vi "Automation.vi"   [LabVIEW 2015]
uses:
  AutomationDriveStates.ctl
  ArmStates.ctl
  <vilib>/Rock Robotics/WPI/Solenoid/WPI_SolenoidValue.ctl
  Robot Global Data.vi
  <vilib>/Rock Robotics/Network Tables/NT Read String.vi
  <vilib>/Rock Robotics/WPI/Solenoid/WPI_SolenoidSetEnum.vi
  <vilib>/addons/control/pid/pid.llb/PID (DBL).vi
  navX-MXP Library/navX-MXP IMU.lvlib
  <vilib>/addons/control/pid/NI_PID_pid.lvlib
types:
  T1 = typedef "AutomationDriveStates.ctl" = enum16{"Find Target", "Just Drive", "Nothing", "Moat", "Rockwall", "Drawbridge Defense", "Drawbridge Drive", "Advance To Defense", "Check Defense Type", "Drive Over Defense", "Stop Drives", "Advance To Target", "Move Forward", "Turn Mid Y", "Move Mid Y", "Center Target"}
  T2 = typedef "ArmStates.ctl" = enum16{"Arm Drive Position", "Winch Up", "Level Arm", "Hold Climb", "Drawbridge Drive Forward", "Shoot Position", "Roll Out", "Hic Up Rollers Off", "Draw Bridge Arm Down", "Harvest Back Down", "Harvest Hic up", "Portcullis", "Sally Door", "Harvest", "Arm Up", "Arm Down"}
  T3 = typedef "WPI_SolenoidValue.ctl" = enum16{"Off", "On", "Forward", "Reverse"}
  T4 = cluster{"proportional gain (Kc)":dbl, "integral time (Ti, min)":dbl, "derivative time (Td, min)":dbl}
  T5 = cluster{"Direction (T=CW)":bool, "Target Left Pos":dbl, "Target Right Pos":dbl, "Target Width":dbl, "Target Center":dbl, "Target Distance from Right":dbl, "Left Drive Speed":dbl, "Right Drive Speed":dbl, "System State":T1, "Lost Target Counter":dbl, "Last Drive Time":u32, "Distance From Target":dbl, "Starting Heading":dbl, "Current Heading":dbl, "Delta Heading":dbl, "Initial Diustance to Target":dbl, "Starting Encoder Position":dbl, "Current Encoder Position":dbl, "Encoder Counts Per Real Ft":dbl, "Encoder Count Per Calc Ft":dbl, "Starting Calc Distance":dbl, "Starting Left Position":dbl, "Starting Right Position":dbl, "Target Angle":dbl, "Target Distance":dbl, "In Position?":bool, "Desired Arm State":T2, "Shoot":bool, "Spin Up Shooter Wheels":bool, "Right of Target":bool, "Drive To Defense Counter":u32}
  T6 = typedef "WPI_MotorControlDeviceRef.ctl" = cluster{"DeviceStatus":errorcluster, "Type":T7, "PWM":cluster{"PWM Channel":T8, "DeadBand":T9}, "CAN":cluster{"Device Number":u8, "Control Mode":T10, "Semaphore":T11, "Max Vout":dbl, "TalonSRX Control Mode":T12}, "Invert":bool}
  T7 = typedef "WPI_MotorControlType.ctl" = enum16{"PWM", "CAN", "CANTalonSRX"}
  T8 = typedef "FPGA_DIOPWMChannel.ctl" = enum8{"PWM 0", "PWM 1", "PWM 2", "PWM 3", "PWM 4", "PWM 5", "PWM 6", "PWM 7", "PWM 8", "PWM 9", "PWM MXP 0", "PWM MXP 1", "PWM MXP 2", "PWM MXP 3", "PWM MXP 4", "PWM MXP 5", "PWM MXP 6", "PWM MXP 7", "PWM MXP 8", "PWM MXP 9", "Invalid"}
  T9 = typedef "WPI_PWMDeadband.ctl" = cluster{"Name":string, "maxPositivePwm":i32, "minPositivePwm":i32, "centerPwm":i32, "maxNegativePwm":i32, "minNegativePwm":i32, "angularRange":u16}
  T10 = typedef "WPI_CANJaguar_ControlMode.ctl" = enum8{"Percent VBus", "Current", "Speed", "Position", "Voltage"}
  T11 = typedef "Semaphore RefNum" = refnum<k1>
  T12 = typedef "WPI_CANTalonSRX_APIControlMode.ctl" = enum8{"Percent VBus", "Speed", "Position", "Slave", "Unchanged / Invalid", "Voltage Compensation", "Current", "Motion Profile"}
  T13 = typedef "navX-MXP IMU.lvlib/navX Device TypeDef.ctl" = cluster{"navX Interface Protocol":T14, "navX Interface Protocol TypeDefs":cluster{"SPIDevRef":T15, "I2CDevRef":T17}, "navX System Information":cluster{"Board Information":T19, "Status":T22, "Offsets":T26, "LastSampleTimestamp":dbl, "LastSampleValid":bool}, "navX Common Information":cluster{"Update Rate (4Hz-60Hz)":T27, "refnum name":string, "error":errorcluster, "LastSampleFPGATimestamp":dbl}}
  T14 = typedef "navX-MXP IMU.lvlib/navX Interface Protocol.ctl" = enum16{"SPI", "I2C", "SERIAL"}
  T15 = typedef "WPI_SPIDevRef.ctl" = cluster{"DevStatus":errorcluster, "Handle":i32, "SPI Bus":T16}
  T16 = typedef "spi_bus.ctl" = enum16{"SPI On-Board, CS0", "SPI On-Board, CS1", "SPI On-Board, CS2", "SPI On-Board, CS3", "SPI MXP", "Invalid"}
  T17 = typedef "WPI_I2CDevRef.ctl" = cluster{"DevStatus":errorcluster, "Device Address":u8, "Handle":i32, "I2C Bus":T18}
  T18 = typedef "i2c_bus.ctl" = enum16{"I2C On-Board", "I2C MXP", "Invalid"}
  T19 = typedef "navX-MXP IMU.lvlib/navX Board Information.ctl" = cluster{"WhoAmI (50 | 0x32)":u8, "Board Revision":u8, "Firmware Major Version":u8, "Firmware Minor Version":u8, "NAVX_BOARD_CAPABILITY":T20, "NAVX_BOARD_YAW_AXIS":T21}
  T20 = typedef "navX-MXP IMU.lvlib/navX NAVX_BOARD_CAPABILITY.ctl" = cluster{"OMNIMOUNT":bool, "YAW_RESET":bool, "VEL_AND_DISP":bool}
  T21 = typedef "navX-MXP IMU.lvlib/navX NAVX_BOARD_YAW_AXIS.ctl" = cluster{"BOARD_YAW_AXIS_UP":bool, "BOARD_YAW_AXIS":u8}
  T22 = typedef "navX-MXP IMU.lvlib/navX Status Data.ctl" = cluster{"Update Rate Hz":u8, "Accelerometer Full-Scale Range":u8, "Gyro Full-Scale Range":u16, "NAVX_OP_STATUS":T23, "NAVX_CAL_STATUS":T24, "NAVX_SELFTEST_STATUS":u8, "NAVX_SENSOR_STATUS":T25}
  T23 = typedef "navX-MXP IMU.lvlib/navX NAVX_OP_STATUS.ctl" = u8
  T24 = typedef "navX-MXP IMU.lvlib/navX NAVX_CAL_STATUS.ctl" = u8
  T25 = typedef "navX-MXP IMU.lvlib/navX NAVX_SENSOR_STATUS.ctl" = cluster{"MOVING":bool, "YAW_STABLE":bool, "MAG_DISTURBANCE":bool, "ALTITUDE_VALID":bool, "SEALEVEL_PRESS_SET":bool, "FUSED_HEADING_VALID":bool}
  T26 = typedef "navX-MXP IMU.lvlib/navX Offsets Data.ctl" = cluster{"Yaw":dbl, "Quat W":dbl, "Quat X":dbl, "Quat Y":dbl, "Quat Z":dbl}
  T27 = typedef "navX-MXP IMU.lvlib/navX Update Rate.ctl" = u8
  T28 = typedef "WPI_CANTalonSRX_GlobalStatus.ctl" = cluster{"Applied Throttle":dbl, "Module Enabled":bool, "CAN Error":errorcluster, "Closed Loop Error":dbl, "Forward Limit Switch Closed":bool, "Reverse Limit Switch Closed":bool, "Sensor Position":dbl, "Sensor Velocity":dbl, "Current":dbl, "Sticky Fault - Over Temp":bool, "Sticky Fault - Under Voltage":bool, "Sticky Fault - Forward Limit":bool, "Sticky Fault - Reverse Limit":bool, "Sticky Fault - Forward Soft Limit":bool, "Sticky Fault - Reverse Soft Limit":bool, "Brake is Enabled":bool, "Encoder Position":dbl, "Encoder Velocity":dbl, "Encoder Index Count":dbl, "Encoder A Pin State":bool, "Encoder B Pin State":bool, "Encoder Index Pin State":bool, "Analog In":dbl, "Analog In Velocity":dbl, "Temperature (C)":dbl, "Battery Voltage":dbl, "Control 5 Is Supported":bool, "Current Profile Slot Select":dbl, "Pos Div 8":bool, "Vel Div 4":bool, "Pulse Width Position":i32, "Pulse Width Velocity":i32, "Pulse Width Rise To Rise (us)":i32, "Pulse Width Rise To Fall (us)":i32, "Mot Prof Active Is Under Run":bool, "Mot Prof Active Has Under Run":bool, "Mot Prof Active Is Last":bool, "Mot Prof Active Velocity Only":bool, "Mot Prof Active Is Valid":bool, "Mot Prof Buffer Is Full":bool, "Mot Prof Active Profile Slot Select":i32, "Mot Prof NextID":i32, "Mot Prof Count":i32, "Mot Prof Active Velocity":dbl, "Mot Prof Active Position":dbl, "Mot Prof Output Enable":i32}
  T29 = typedef "navX-MXP IMU.lvlib/navX YPRH Data.ctl" = cluster{"Yaw":dbl, "Pitch":dbl, "Roll":dbl, "Heading":dbl}
  T30 = typedef "WPI_SolenoidDevRef.ctl" = cluster{"DevStatus":errorcluster, "Pneumatics Control Module":u8, "Forward Solenoid Channel":T31, "Reverse Solenoid Channel":T31}
  T31 = typedef "WPI_SolenoidChannel.ctl" = enum8{"Solenoid 0", "Solenoid 1", "Solenoid 2", "Solenoid 3", "Solenoid 4", "Solenoid 5", "Solenoid 6", "Solenoid 7", "Invalid"}
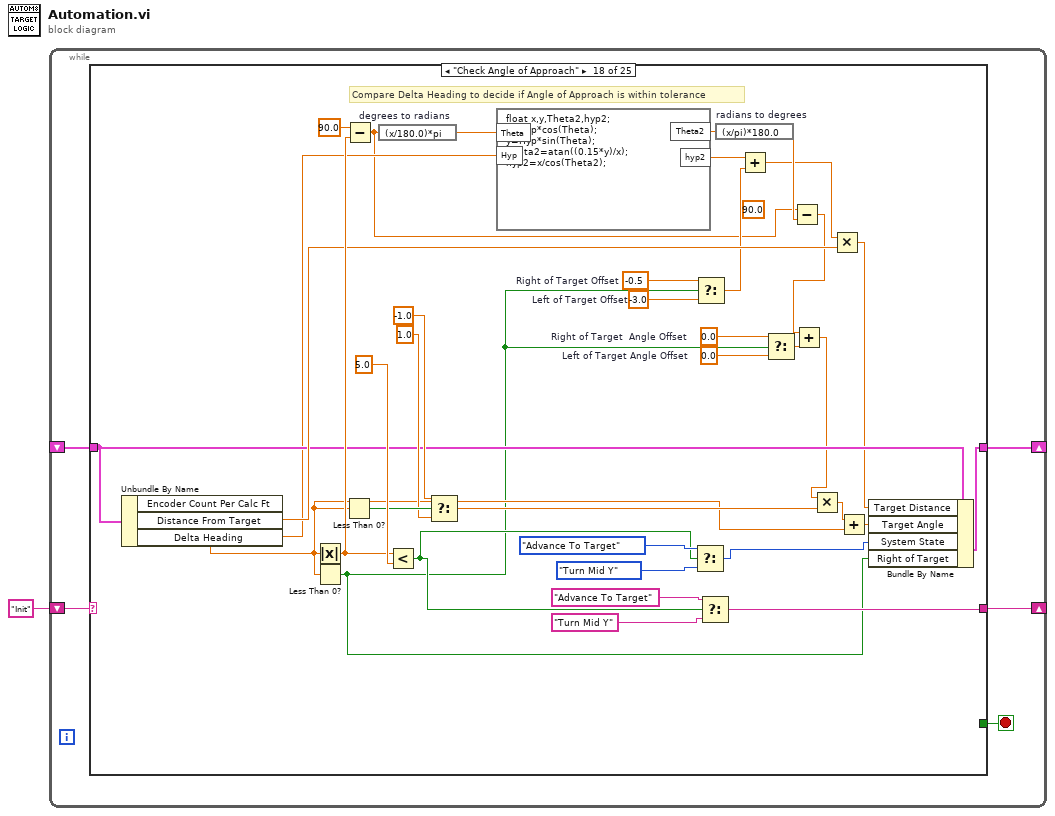
[diagram p0: block diagram]
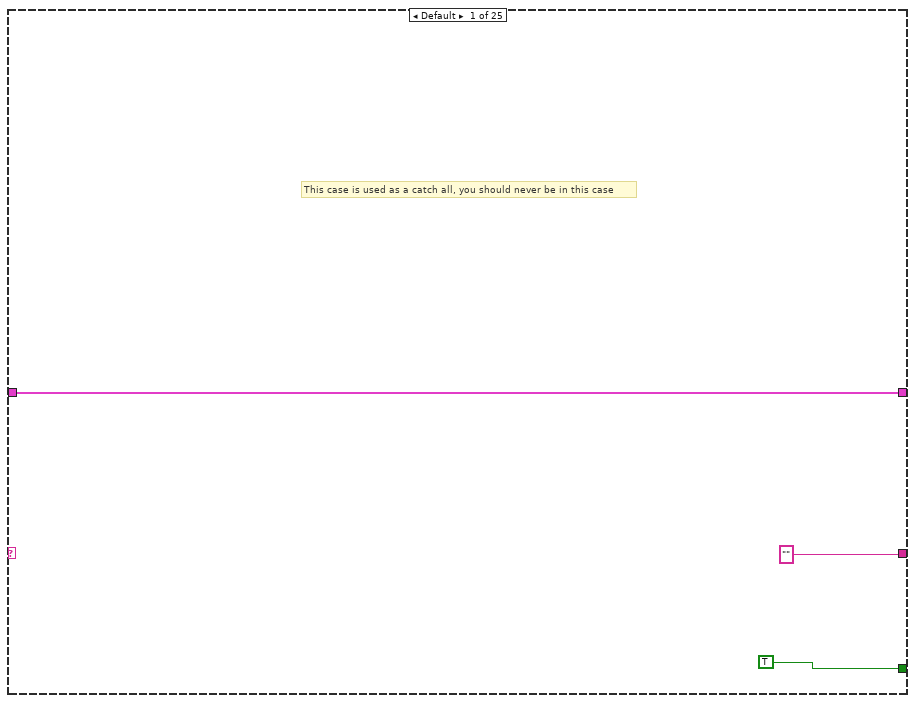
[diagram p2: hidden frame]
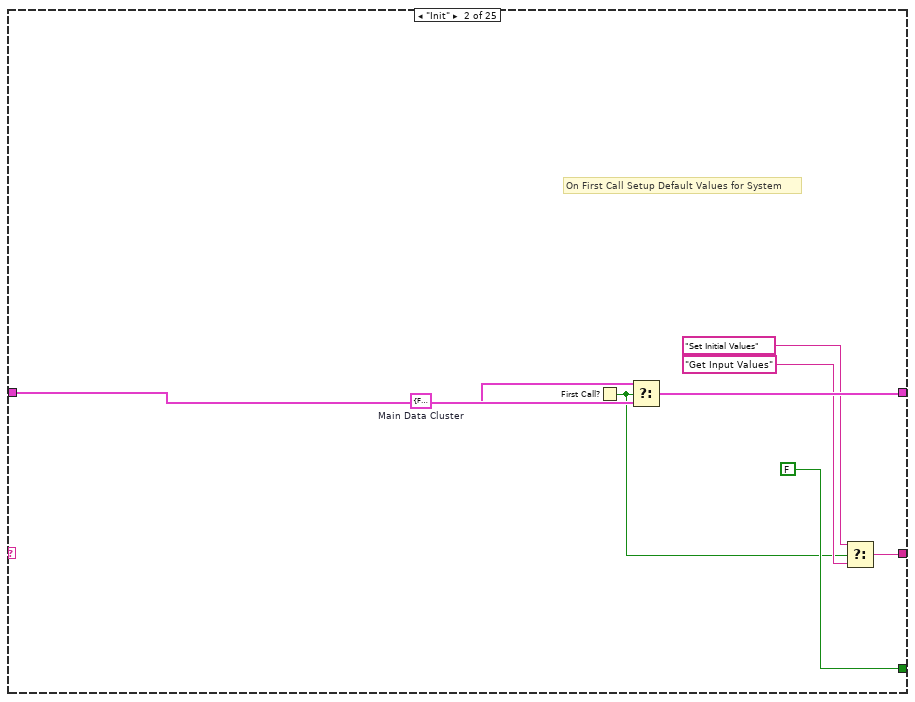
[diagram p3: hidden frame]
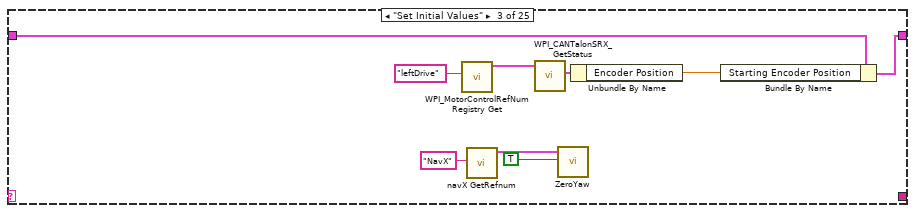
[diagram p4: hidden frame]
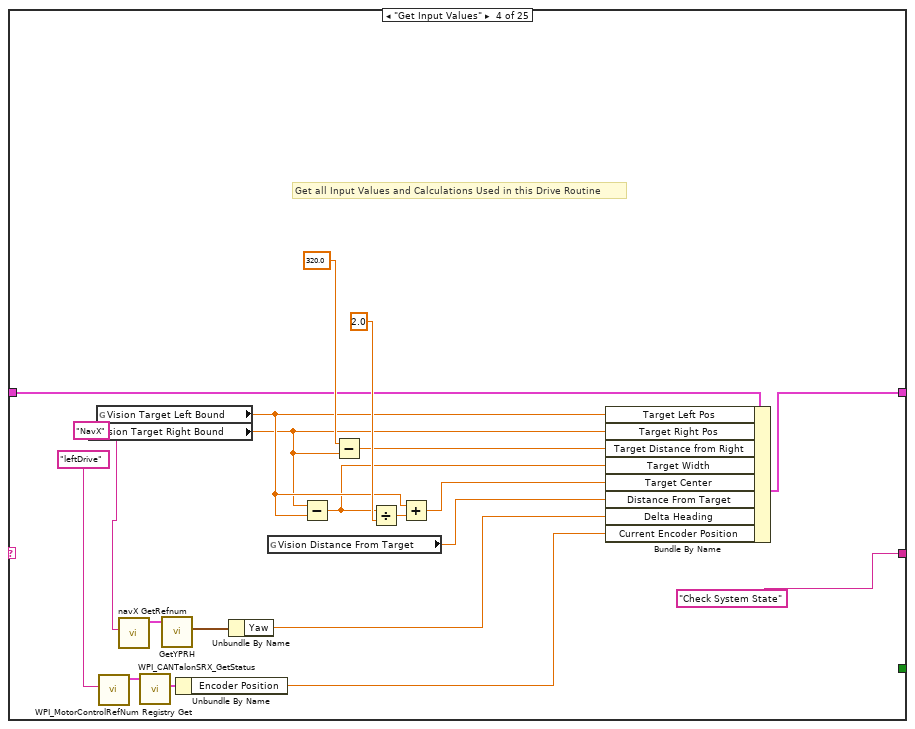
[diagram p5: hidden frame]
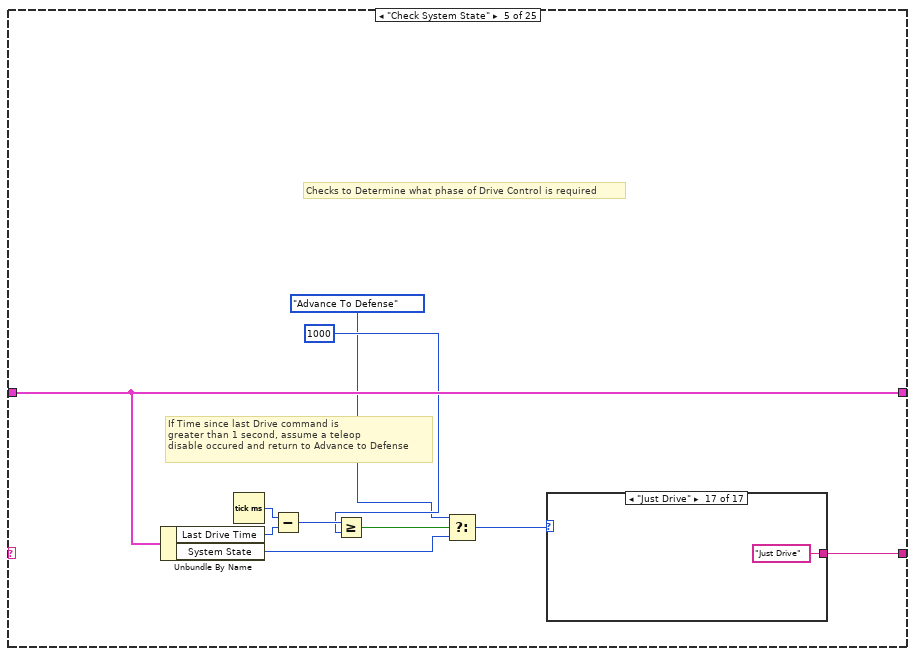
[diagram p6: hidden frame]
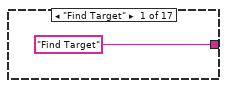
[diagram p7: hidden frame]
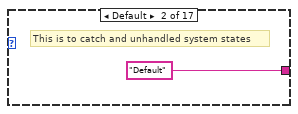
[diagram p8: hidden frame]
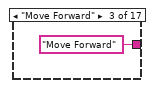
[diagram p9: hidden frame]
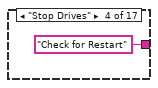
[diagram p10: hidden frame]
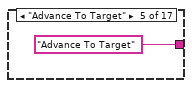
[diagram p11: hidden frame]
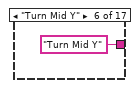
[diagram p12: hidden frame]
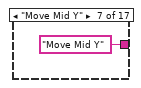
[diagram p13: hidden frame]
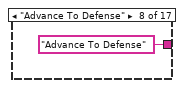
[diagram p14: hidden frame]
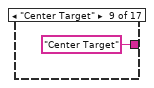
[diagram p15: hidden frame]
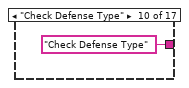
[diagram p16: hidden frame]
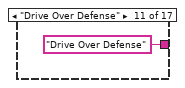
[diagram p17: hidden frame]
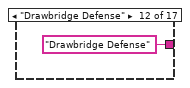
[diagram p18: hidden frame]
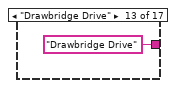
[diagram p19: hidden frame]
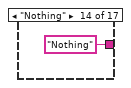
[diagram p20: hidden frame]
diagram:
  n1 = while {
    shift-right: [w6] -> _
    shift-left: "Init" -> [w2]
    shift-right: [w5] -> _
    shift-left: _ -> [w4]
    stop <- w3 stop-if-true
    n2 = case shown="\"Check Angle of Approach\"" w2 {
      tunnel: ["" w10 _ "Check System State" w55 w75 w108 w127 w144 "Drive Motors" w166 w183 w197 w215 w248 "Drive Motors" w287 w330 w343 w366 "Check for Stop" w407 "Exit" "Exit" _] -> w6
      tunnel: [w9 w14 w25 w43 w56 w102 w113 w135 w152 w157 w174 w191 w206 w210 w254 w277 w299 w329 w355 w374 w403 w411 w438 w483 w500] -> w5
      tunnel: w4 -> [w9 w16 w26 w36 w56 w100 w112 w133 w150 w155 w172 w189 w193 w211 w255 w278 w297 w318 w356 w372 w404 w412 w437 w484 w500]
      tunnel: [TRUE FALSE _ _ _ _ _ _ _ _ _ _ _ _ _ _ _ _ _ _ _ _ _ _ TRUE] -> w3
      frame Default {
        # "This case is used as a catch all, you should never be in this case"
      }
      frame "Init" {
        w15 = T5 {"Direction (T=CW)"=FALSE, "Target Left Pos"=0.0, "Target Right Pos"=0.0, "Target Width"=0.0, "Target Center"=0.0, "Target Distance from Right"=0.0, "Left Drive Speed"=0.0, "Right Drive Speed"=0.0, "System State"=enum."Advance To Defense", "Lost Target Counter"=0.0, "Last Drive Time"=0, "Distance From Target"=0.0, "Starting Heading"=0.0, "Current Heading"=0.0, "Delta Heading"=0.0, "Initial Diustance to Target"=0.0, "Starting Encoder Position"=0.0, "Current Encoder Position"=0.0, "Encoder Counts Per Real Ft"=0.0, "Encoder Count Per Calc Ft"=0.0, "Starting Calc Distance"=0.0, "Starting Left Position"=0.0, "Starting Right Position"=0.0, "Target Angle"=0.0, "Target Distance"=0.0, "In Position?"=FALSE, "Desired Arm State"=enum."Arm Drive Position", "Shoot"=FALSE, "Spin Up Shooter Wheels"=FALSE, "Right of Target"=FALSE, "Drive To Defense Counter"=0}  # Main Data Cluster
        # "On First Call Setup Default Values for System"
        n3 = First Call?() -> (First Call?: T/F=w11:bool)
        n4 = Select(t=w15, s=w11, f=w16) -> (s? t:f=w14:T5)
        n5 = Select(t="Set Initial Values", s=w11, f="Get Input Values") -> (s? t:f=w10:string)
      }
      frame "Set Initial Values" {
        n6 = call <vilib>:"WPI_MotorControlRefNum Registry Get.vi"("refnum name"="leftDrive") -> ("MotorControlDevRef"=w24:T6)  [unwired: 9 in, 1 out]
        n7 = call "navX GetRefnum.vi"("refnum name"="NavX") -> ("navX Device TypeDef"=w20:T13)  [unwired: 9 in, 1 out]
        n8 = call <vilib>:"WPI_CANTalonSRX_GetStatus.vi"("CAN Talon SRX Ref"=w24) -> ("Talon SRX Status"=w23:T28)  [unwired: 8 in, 2 out]
        n9 = call "ZeroYaw.vi"("Reset(F)"=TRUE, "navX Device TypeDef"=w20) -> ()  [unwired: 8 in, 2 out]
        n10 = Unbundle By Name(w23) -> ("Encoder Position"=w21:dbl)
        n11 = Bundle By Name(cluster=w26, "Starting Encoder Position"=w21) -> (w25:T5)
      }
      frame "Get Input Values" {
        # "Get all Input Values and Calculations Used in this Drive Routine"
        n12 = global read "Robot Global Data.vi" "Vision Target Right Bound"() -> (w41:dbl)
        n13 = global read "Robot Global Data.vi" "Vision Target Left Bound"() -> (w42:dbl)
        n14 = call <vilib>:"WPI_MotorControlRefNum Registry Get.vi"("refnum name"="leftDrive") -> ("MotorControlDevRef"=w33:T6)  [unwired: 9 in, 1 out]
        n15 = call "navX GetRefnum.vi"("refnum name"="NavX") -> ("navX Device TypeDef"=w30:T13)  [unwired: 9 in, 1 out]
        n16 = call <vilib>:"WPI_CANTalonSRX_GetStatus.vi"("CAN Talon SRX Ref"=w33) -> ("Talon SRX Status"=w32:T28)  [unwired: 8 in, 2 out]
        n17 = call "GetYPRH.vi"("navX Device TypeDef"=w30) -> ("YPRH"=w29:T29)  [unwired: 8 in, 2 out]
        n18 = Unbundle By Name(w32) -> ("Encoder Position"=w31:dbl)
        n19 = Unbundle By Name(w29) -> ("Yaw"=w28:dbl)
        n20 = global read "Robot Global Data.vi" "Vision Distance From Target"() -> (w37:dbl)
        n21 = Subtract(x=w41, y=w42) -> (x-y=w39:dbl)
        n22 = Subtract(x=320.0, y=w41) -> (x-y=w40:dbl)
        n23 = Divide(x=w39, y=2.0) -> (x/y=w45:dbl)
        n24 = Add(x=w42, y=w45) -> (x+y=w38:dbl)
        n25 = Bundle By Name(cluster=w36, "Target Left Pos"=w42, "Target Right Pos"=w41, "Target Distance from Right"=w40, "Target Width"=w39, "Target Center"=w38, "Distance From Target"=w37, "Delta Heading"=w28, "Current Encoder Position"=w31) -> (w43:T5)
      }
      frame "Check System State" {
        # "If Time since last Drive command is\ngreater than 1 second, assume a teleop\ndisable occured and return to Advance to Defense"
        # "Checks to Determine what phase of Drive Control is required"
        n26 = Unbundle By Name(w56) -> ("Last Drive Time"=w54:u32, "System State"=w49:T1)
        n27 = Tick Count (ms)() -> (millisecond timer value=w53:u32)
        n28 = Subtract(x=w53, y=w54) -> (x-y=w52:u32)
        n29 = Greater Or Equal?(x=w52, y=u32 1000) -> (x >= y?=w48:bool)
        n30 = Select(t=AutomationDriveStates."Advance To Defense", s=w48, f=w49) -> (s? t:f=w50:T1)
        n31 = case shown="\"Just Drive\"" w50 {
          tunnel: ["Find Target" "Default" "Move Forward" "Check for Restart" "Advance To Target" "Turn Mid Y" "Move Mid Y" "Advance To Defense" "Center Target" "Check Defense Type" "Drive Over Defense" "Drawbridge Defense" "Drawbridge Drive" "Nothing" "Moat" "Rockwall" "Just Drive"] -> w55
          frame "Find Target" {
          }
          frame Default {
            # "This is to catch and unhandled system states"
          }
          frame "Move Forward" {
          }
          frame "Stop Drives" {
          }
          frame "Advance To Target" {
          }
          frame "Turn Mid Y" {
          }
          frame "Move Mid Y" {
          }
          frame "Advance To Defense" {
          }
          frame "Center Target" {
          }
          frame "Check Defense Type" {
          }
          frame "Drive Over Defense" {
          }
          frame "Drawbridge Defense" {
          }
          frame "Drawbridge Drive" {
          }
          frame "Nothing" {
          }
          frame "Moat" {
          }
          frame "Rockwall" {
          }
          frame "Just Drive" {
          }
        }
      }
      frame "Advance To Defense" {
        w101 = 0.55 ("Left Drive Speed")
        # "Using constants based on visual data"
        # "Moving the Robot to Start of Defense"
        n32 = Unbundle By Name(w100) -> ("Drive To Defense Counter"=w85:u32, "Starting Encoder Position"=w99:dbl, "Current Encoder Position"=w98:dbl)  [unwired: 1 out]
        n33 = Subtract(x=w99, y=w98) -> (x-y=w97:dbl)
        n34 = Absolute Value(x=w97) -> (abs(x)=w94:dbl)
        n35 = Multiply(x=456.0 ("Encoder Counts Per Real Ft"), y=4.5) -> (x*y=w90:dbl)
        n36 = Increment(x=w85) -> (x+1=w84:u32)
        n37 = Greater Or Equal?(x=w94, y=w90) -> (x >= y?=w80:bool)
        n38 = Greater?(x=w84, y=u32 50) -> (0:w81:bool)
        n39 = Or(x=w81, y=w80) -> (x .or. y?=w82:bool)
        n40 = call-poly <vilib>:"NT Read Value.vi"("Name"="Auto Selector") -> ("String"=w74:string)  [unwired: 9 in, 1 out]
        n41 = Select(t=AutomationDriveStates."Check Defense Type" ("System State"), s=w82, f=AutomationDriveStates."Advance To Defense" ("System State")) -> (s? t:f=w78:T1)
        n42 = case shown="\"Nothing\"" w74 {
          tunnel: [w105 AutomationDriveStates."Nothing" ("System State")] -> w77
          tunnel: w78 -> [w105 _]
          frame Default {
          }
          frame "Nothing" {
          }
        }
        n43 = Select(t="Check Defense Type", s=w82, f="Drive Motors") -> (s? t:f=w76:string)
        n44 = case shown="\"Nothing\"" w74 {
          tunnel: [w103 "Nothing"] -> w75
          tunnel: w76 -> [w103 _]
          frame Default {
          }
          frame "Nothing" {
          }
        }
        n45 = Bundle By Name(cluster=w100, "Drive To Defense Counter"=w84, "Left Drive Speed"=w101, "Right Drive Speed"=w101, "System State"=w77, "Desired Arm State"=ArmStates."Portcullis", "Shoot"=FALSE, "Spin Up Shooter Wheels"=FALSE) -> (w102:T5)
      }
      frame "Check Defense Type" {
        n46 = Unbundle By Name(w112) -> ("Current Encoder Position"=w111:dbl)
        n47 = call-poly <vilib>:"NT Read Value.vi"("Name"="Auto Selector") -> ("String"=w109:string)  [unwired: 9 in, 1 out]
        n48 = case shown="\"Just Drive\"" w109 {
          tunnel: [AutomationDriveStates."Drive Over Defense" ("System State") AutomationDriveStates."Moat" ("System State") AutomationDriveStates."Drawbridge Defense" ("System State") AutomationDriveStates."Rockwall" ("System State") AutomationDriveStates."Just Drive" ("System State")] -> w107
          frame "Drive Over", Default {
          }
          frame "Moat" {
          }
          frame "Drawbridge" {
          }
          frame "Rockwall" {
          }
          frame "Just Drive" {
          }
        }
        n49 = Bundle By Name(cluster=w112, "System State"=w107, "Starting Encoder Position"=w111) -> (w113:T5)
        n50 = Format Into String(w107) -> (resulting string=w108:string)  [unwired: 3 in, 1 out]
      }
      frame "Drive Over Defense" {
        w134 = 1.0 ("Left Drive Speed")
        # "Was 5.5 feet"
        # "Using constants based on visual data"
        # "Moving the Robot to Start of Defense"
        n51 = Unbundle By Name(w133) -> ("Starting Encoder Position"=w132:dbl, "Current Encoder Position"=w131:dbl)
        n52 = Subtract(x=w132, y=w131) -> (x-y=w130:dbl)
        n53 = Absolute Value(x=w130) -> (abs(x)=w126:dbl)
        n54 = Multiply(x=456.0 ("Encoder Counts Per Real Ft"), y=8.0) -> (x*y=w120:dbl)
        n55 = Greater Or Equal?(x=w126, y=w120) -> (x >= y?=w122:bool)
        n56 = Select(t="Find Target", s=w122, f="Drive Motors") -> (s? t:f=w127:string)
        n57 = Select(t=AutomationDriveStates."Find Target" ("System State"), s=w122, f=AutomationDriveStates."Drive Over Defense" ("System State")) -> (s? t:f=w123:T1)
        n58 = Bundle By Name(cluster=w133, "Left Drive Speed"=w134, "Right Drive Speed"=w134, "System State"=w123) -> (w135:T5)
      }
      frame "Just Drive" {
        w151 = 1.0 ("Left Drive Speed")
        # "Was 5.5 feet"
        # "Using constants based on visual data"
        # "Moving the Robot to Start of Defense"
        n59 = Unbundle By Name(w150) -> ("Starting Encoder Position"=w149:dbl, "Current Encoder Position"=w148:dbl)
        n60 = Subtract(x=w149, y=w148) -> (x-y=w147:dbl)
        n61 = Absolute Value(x=w147) -> (abs(x)=w143:dbl)
        n62 = Multiply(x=456.0 ("Encoder Counts Per Real Ft"), y=10.0) -> (x*y=w138:dbl)
        n63 = Greater Or Equal?(x=w143, y=w138) -> (x >= y?=w140:bool)
        n64 = Select(t="Nothing", s=w140, f="Drive Motors") -> (s? t:f=w144:string)
        n65 = Select(t=AutomationDriveStates."Nothing" ("System State"), s=w140, f=AutomationDriveStates."Just Drive" ("System State")) -> (s? t:f=w141:T1)
        n66 = Bundle By Name(cluster=w150, "Left Drive Speed"=w151, "Right Drive Speed"=w151, "System State"=w141) -> (w152:T5)
      }
      frame "Nothing" {
        w156 = 0.0 ("Left Drive Speed")
        # "Using constants based on visual data"
        # "Moving the Robot to Start of Defense"
        n67 = Bundle By Name(cluster=w155, "Left Drive Speed"=w156, "Right Drive Speed"=w156, "System State"=AutomationDriveStates."Nothing") -> (w157:T5)
      }
      frame "Moat" {
        w173 = 1.0 ("Left Drive Speed")
        # "Using constants based on visual data"
        # "Moving the Robot to Start of Defense"
        n68 = Unbundle By Name(w172) -> ("Starting Encoder Position"=w171:dbl, "Current Encoder Position"=w170:dbl)
        n69 = Subtract(x=w171, y=w170) -> (x-y=w169:dbl)
        n70 = Absolute Value(x=w169) -> (abs(x)=w165:dbl)
        n71 = Multiply(x=456.0 ("Encoder Counts Per Real Ft"), y=12.0) -> (x*y=w159:dbl)
        n72 = Greater Or Equal?(x=w165, y=w159) -> (x >= y?=w161:bool)
        n73 = Select(t="Find Target", s=w161, f="Drive Motors") -> (s? t:f=w166:string)
        n74 = Select(t=AutomationDriveStates."Find Target" ("System State"), s=w161, f=AutomationDriveStates."Moat" ("System State")) -> (s? t:f=w162:T1)
        n75 = Bundle By Name(cluster=w172, "Left Drive Speed"=w173, "Right Drive Speed"=w173, "System State"=w162) -> (w174:T5)
      }
      frame "Rockwall" {
        w190 = 1.0 ("Left Drive Speed")
        # "Using constants based on visual data"
        # "Moving the Robot to Start of Defense"
        n76 = Unbundle By Name(w189) -> ("Starting Encoder Position"=w188:dbl, "Current Encoder Position"=w187:dbl)
        n77 = Subtract(x=w188, y=w187) -> (x-y=w186:dbl)
        n78 = Absolute Value(x=w186) -> (abs(x)=w182:dbl)
        n79 = Multiply(x=456.0 ("Encoder Counts Per Real Ft"), y=10.0) -> (x*y=w176:dbl)
        n80 = Greater Or Equal?(x=w182, y=w176) -> (x >= y?=w178:bool)
        n81 = Select(t="Find Target", s=w178, f="Drive Motors") -> (s? t:f=w183:string)
        n82 = Select(t=AutomationDriveStates."Find Target" ("System State"), s=w178, f=AutomationDriveStates."Rockwall" ("System State")) -> (s? t:f=w179:T1)
        n83 = Bundle By Name(cluster=w189, "Left Drive Speed"=w190, "Right Drive Speed"=w190, "System State"=w179) -> (w191:T5)
      }
      frame "Drawbridge Defense" {
        n84 = Unbundle By Name(w193) -> ("Current Encoder Position"=w192:dbl)
        n85 = global read "Robot Global Data.vi" "Arm State"() -> (w202:T2)
        n86 = Equal?(x=w202, y=ArmStates."Arm Drive Position" ("Desired Arm State")) -> (x = y?=w194:bool)
        n87 = global read "Robot Global Data.vi" "Right Drive Overide"() -> (w205:dbl)
        n88 = global read "Robot Global Data.vi" "Left Drive Overide"() -> (w204:dbl)
        n89 = Select(t=AutomationDriveStates."Drawbridge Drive" ("System State"), s=w194, f=AutomationDriveStates."Drawbridge Defense" ("System State")) -> (s? t:f=w199:T1)
        n90 = Bundle By Name(cluster=w193, "Starting Encoder Position"=w192, "Right Drive Speed"=w205, "Left Drive Speed"=w204, "Desired Arm State"=ArmStates."Draw Bridge Arm Down", "System State"=w199) -> (w206:T5)
        n91 = Select(t="Drawbridge Drive", s=w194, f="Drive Motors") -> (s? t:f=w197:string)
      }
      frame "Drawbridge Drive" {
        w207 = 0.4 ("Left Drive Speed")
        n92 = Unbundle By Name(w211) -> ("Starting Encoder Position"=w222:dbl, "Current Encoder Position"=w221:dbl)
        n93 = Subtract(x=w222, y=w221) -> (x-y=w220:dbl)
        n94 = Absolute Value(x=w220) -> (abs(x)=w219:dbl)
        n95 = Multiply(x=456.0, y=9.0) -> (x*y=w218:dbl)
        n96 = Greater?(x=w219, y=w218) -> (0:w208:bool)
        n97 = Select(t=AutomationDriveStates."Find Target" ("System State"), s=w208, f=AutomationDriveStates."Drive Over Defense" ("System State")) -> (s? t:f=w209:T1)
        n98 = Bundle By Name(cluster=w211, "System State"=w209, "Left Drive Speed"=w207, "Right Drive Speed"=w207) -> (w210:T5)
        n99 = Select(t="Find Target", s=w208, f="Drive Motors") -> (s? t:f=w215:string)
      }
      frame "Find Target" {
        w227 = 0.45  # In Position Speed
        w228 = 0.4  # Initial Find Target Speed
        # "Used to Determine the Rotational Speed and Direction of the Robot to find the center of target"
        n100 = Unbundle By Name(w255) -> ("Delta Heading"=w242:dbl, "Target Center"=w246:dbl, "Current Encoder Position"=w239:dbl, "Distance From Target"=w238:dbl, "In Position?"=w224:bool, "Target Left Pos"=w237:dbl, "Target Right Pos"=w236:dbl)
        n101 = Less Or Equal To 0?(x=w242) -> (x <= 0?=w241:bool)
        n102 = Equal To 0?(x=w246) -> (x = 0?=w244:bool)
        n103 = Greater?(x=w246, y=160) -> (0:w243:bool)
        n104 = In Range and Coerce(upper limit=170 ("lower limit"), x=w246, lower limit=150) -> (In Range?=w240:bool)  [unwired: 1 out]
        n105 = Select(t=w227, s=w224, f=w228) -> (s? t:f=w225:dbl)
        n106 = Select(t=w241, s=w244, f=w243) -> (s? t:f=w245:bool)
        n107 = Negate(x=w225) -> (-x=w226:dbl)
        n108 = Select(t="Advance To Target", s=w224, f="Move Forward") -> (s? t:f=w231:string)
        n109 = Select(t=AutomationDriveStates."Advance To Target" ("System State"), s=w224, f=AutomationDriveStates."Move Forward" ("System State")) -> (s? t:f=w233:T1)
        n110 = Select(t=w233, s=w240, f=AutomationDriveStates."Find Target" ("System State")) -> (s? t:f=w250:T1)
        n111 = Select(t=w231, s=w240, f="Drive Motors") -> (s? t:f=w248:string)
        n112 = Select(t=w225, s=w245, f=w226) -> (s? t:f=w253:dbl)
        n113 = Select(t=w226, s=w245, f=w225) -> (s? t:f=w252:dbl)
        n114 = Bundle By Name(cluster=w255, "Left Drive Speed"=w253, "Right Drive Speed"=w252, "Direction (T=CW)"=w245, "System State"=w250, "Starting Encoder Position"=w239, "Starting Calc Distance"=w238, "Starting Left Position"=w237, "Starting Right Position"=w236, "Desired Arm State"=ArmStates."Shoot Position") -> (w254:T5)
      }
      frame "Center Target" {
        w263 = 0.2  # Center Target Speed
        # "Used to Determine the Rotational Speed and Direction of the Robot to find the center of target"
        n115 = Unbundle By Name(w278) -> ("Delta Heading"=w267:dbl, "Target Center"=w271:dbl)
        n116 = Less Or Equal To 0?(x=w267) -> (x <= 0?=w266:bool)
        n117 = Equal To 0?(x=w271) -> (x = 0?=w269:bool)
        n118 = Greater?(x=w271, y=160) -> (0:w268:bool)
        n119 = In Range and Coerce(upper limit=165 ("lower limit"), x=w271, lower limit=155) -> (In Range?=w258:bool)  [unwired: 1 out]
        n120 = Select(t=w266, s=w269, f=w268) -> (s? t:f=w270:bool)
        n121 = Negate(x=w263) -> (-x=w265:dbl)
        n122 = Select(t=AutomationDriveStates."Stop Drives" ("System State"), s=w258, f=AutomationDriveStates."Center Target" ("System State")) -> (s? t:f=w273:T1)
        n123 = Select(t=TRUE, s=w258, f=FALSE) -> (s? t:f=w259:bool)
        n124 = Select(t=w263, s=w270, f=w265) -> (s? t:f=w276:dbl)
        n125 = Select(t=w265, s=w270, f=w263) -> (s? t:f=w275:dbl)
        n126 = Bundle By Name(cluster=w278, "Left Drive Speed"=w276, "Right Drive Speed"=w275, "Direction (T=CW)"=w270, "System State"=w273, "Shoot"=w259) -> (w277:T5)
      }
      frame "Move Forward" {
        (unwired) 815.0 ("Encoder Count Per Calc Ft")
        w298 = 0.0 ("Left Drive Speed")
        # "Moving the Robot 1 ft closer to target"
        n127 = Unbundle By Name(w297) -> ("Target Center"=w290:dbl, "Starting Encoder Position"=w296:dbl, "Current Encoder Position"=w283:dbl, "Starting Calc Distance"=w292:dbl, "Distance From Target"=w291:dbl)  [unwired: 1 out]
        n128 = Subtract(x=w292, y=w291) -> (x-y=w293:dbl)
        n129 = Subtract(x=w296, y=w283) -> (x-y=w295:dbl)
        n130 = Absolute Value(x=w295) -> (abs(x)=w286:dbl)
        n131 = Absolute Value(x=w293) -> (abs(x)=w285:dbl)
        n132 = Greater Than 0?(x=w290) -> (x > 0?=w282:bool)
        n133 = Divide(x=w286, y=w285) -> ()  [unwired: 1 out]
        n134 = Greater Or Equal?(x=w285, y=1.0) -> (x >= y?=w294:bool)
        n135 = Compound Arithmetic op=AND(w282, w294) -> ()  [unwired: 1 out]
        n136 = Bundle By Name(cluster=w297, "Left Drive Speed"=w298, "Right Drive Speed"=w298, "Encoder Count Per Calc Ft"=456.0) -> (w299:T5)
        n137 = Select(t="Check Angle of Approach", s=w282, f="Drive Motors") -> (s? t:f=w287:string)
      }
      frame "Check Angle of Approach" {
        w302 = 0.0  # Left of Target Angle Offset
        w303 = 0.0  # Right of Target  Angle Offset
        w306 = -3.0  # Left of Target Offset
        w307 = -0.5  # Right of Target Offset
        (unwired) 90.0 ("f")
        # "Compare Delta Heading to decide if Angle of Approach is within tolerance"
        n138 = Unbundle By Name(w318) -> ("Encoder Count Per Calc Ft"=w321:dbl, "Distance From Target"=w312:dbl, "Delta Heading"=w311:dbl)
        n139 = Absolute Value(x=w311) -> (abs(x)=w323:dbl)
        n140 = Less Than 0?(x=w311) -> (x < 0?=w301:bool)
        n141 = Less Than 0?(x=w311) -> (x < 0?=w327:bool)
        n142 = Subtract(x=90.0 ("f"), y=w323) -> (x-y=w300:dbl)
        n143 = expression code="(x/180.0)*pi" "degrees to radians"(w300) -> (w317:dbl)
        n144 = Less?(x=w323, y=5.0) -> (x < y?=w331:bool)
        n145 = Select(t=-1.0, s=w327, f=1.0) -> (s? t:f=w322:dbl)
        n146 = formula code="float x,y,Theta2,hyp2;\nx=Hyp*cos(Theta);\ny=Hyp*sin(Theta);\nTheta2=atan((0.15*y)/x);\nhyp2=x/cos(Theta2);"("Theta"=w317, "Hyp"=w312) -> ("Theta2"=w316:dbl, "hyp2"=w310:dbl)
        n147 = Select(t=AutomationDriveStates."Advance To Target" ("System State"), s=w331, f=AutomationDriveStates."Turn Mid Y" ("System State")) -> (s? t:f=w328:T1)
        n148 = Select(t=w307, s=w301, f=w306) -> (s? t:f=w308:dbl)
        n149 = Select(t="Advance To Target", s=w331, f="Turn Mid Y") -> (s? t:f=w330:string)
        n150 = expression code="(x/pi)*180.0" "radians to degrees"(w316) -> (w314:dbl)
        n151 = Add(x=w310, y=w308) -> (x+y=w309:dbl)
        n152 = Select(t=w303, s=w301, f=w302) -> (s? t:f=w304:dbl)
        n153 = Subtract(x=w300, y=w314) -> (x-y=w313:dbl)
        n154 = Add(x=w313, y=w304) -> (x+y=w305:dbl)
        n155 = Multiply(x=w305, y=w322) -> (x*y=w320:dbl)
        n156 = Multiply(x=w309, y=w321) -> (x*y=w315:dbl)
        n157 = Add(x=w320, y=w311) -> (x+y=w319:dbl)
        n158 = Bundle By Name(cluster=w318, "Target Distance"=w315, "Target Angle"=w319, "System State"=w328, "Right of Target"=w301) -> (w329:T5)
      }
      frame "Turn Mid Y" {
        w349 = 5.0
        w357 = -0.5
        w358 = 0.5
        n159 = Unbundle By Name(w356) -> ("Current Encoder Position"=w341:dbl, "Target Angle"=w338:dbl, "Delta Heading"=w337:dbl)
        n160 = Add(x=w338, y=w349) -> (x+y=w351:dbl)
        n161 = Subtract(x=w338, y=w349) -> (x-y=w350:dbl)
        n162 = Max & Min(x=w351, y=w350) -> (max(x,y)=w339:dbl, min(x,y)=w352:dbl)
        n163 = Greater?(x=w338, y=w337) -> (0:w344:bool)
        n164 = In Range and Coerce(upper limit=w339, x=w337, lower limit=w352) -> (In Range?=w340:bool)  [unwired: 1 out]
        n165 = Select(t=w358, s=w344, f=w357) -> (s? t:f=w354:dbl)
        n166 = Select(t=w357, s=w344, f=w358) -> (s? t:f=w353:dbl)
        n167 = Select(t=AutomationDriveStates."Move Mid Y" ("System State"), s=w340, f=AutomationDriveStates."Turn Mid Y" ("System State")) -> (s? t:f=w342:T1)
        n168 = Select(t="Move Mid Y", s=w340, f="Drive Motors") -> (s? t:f=w343:string)
        n169 = Bundle By Name(cluster=w356, "Starting Encoder Position"=w341, "Left Drive Speed"=w354, "Right Drive Speed"=w353, "System State"=w342) -> (w355:T5)
      }
      frame "Move Mid Y" {
        w373 = 0.5 ("Left Drive Speed")
        # "Moving the Robot to Mid Y"
        n170 = Unbundle By Name(w372) -> ("Starting Encoder Position"=w371:dbl, "Current Encoder Position"=w370:dbl, "Target Distance"=w364:dbl)
        n171 = Subtract(x=w371, y=w370) -> (x-y=w369:dbl)
        n172 = Absolute Value(x=w369) -> (abs(x)=w365:dbl)
        n173 = Greater Or Equal?(x=w365, y=w364) -> (x >= y?=w360:bool)
        n174 = Select(t=AutomationDriveStates."Find Target" ("System State"), s=w360, f=AutomationDriveStates."Move Mid Y" ("System State")) -> (s? t:f=w361:T1)
        n175 = Select(t="Find Target", s=w360, f="Drive Motors") -> (s? t:f=w366:string)
        n176 = Bundle By Name(cluster=w372, "Left Drive Speed"=w373, "Right Drive Speed"=w373, "In Position?"=w360, "System State"=w361, "Spin Up Shooter Wheels"=TRUE) -> (w374:T5)
      }
      frame "Advance To Target" {
        w378 = 200.0 ("upper limit")
        w379 = 0.0 ("lower limit")
        w382 = 50.0 ("y")
        w405 = 0.0045 ("y")
        # "If Target is lost for 10 consecutive iterations then return\nto Find Target State"
        # "Used to Calculate Drive Speed of Robot Towards the Target"
        n177 = Unbundle By Name(w404) -> ("Left Drive Speed"=w386:dbl, "Right Drive Speed"=w385:dbl, "Target Left Pos"=w384:dbl, "Target Distance from Right"=w383:dbl, "Lost Target Counter"=w398:dbl, "Target Center"=w402:dbl)
        n178 = Subtract(x=w384, y=w382) -> (x-y=w380:dbl)
        n179 = Subtract(x=w383, y=w382) -> (x-y=w381:dbl)
        n180 = In Range and Coerce(upper limit=w378, x=w381, lower limit=w379) -> (coerced(x)=w376:dbl)  [unwired: 1 out]
        n181 = In Range and Coerce(upper limit=w378, x=w380, lower limit=w379) -> (coerced(x)=w377:dbl)  [unwired: 1 out]
        n182 = Equal To 0?(x=w402) -> (x = 0?=w388:bool)
        n183 = Increment(x=w398) -> (x+1=w399:dbl)
        n184 = Select(t=w399, s=w388, f=0.0) -> (s? t:f=w397:dbl)
        n185 = Multiply(x=w377, y=w405) -> (x*y=w389:dbl)
        n186 = Multiply(x=w405, y=w376) -> (x*y=w391:dbl)
        n187 = Greater Or Equal?(x=w397, y=15.0) -> (x >= y?=w396:bool)
        n188 = Select(t=w386, s=w388, f=w389) -> (s? t:f=w387:dbl)
        n189 = Select(t=w385, s=w388, f=w391) -> (s? t:f=w390:dbl)
        n190 = Select(t=AutomationDriveStates."Find Target" ("System State"), s=w396, f=AutomationDriveStates."Advance To Target" ("System State")) -> (s? t:f=w394:T1)
        n191 = Bundle By Name(cluster=w404, "Left Drive Speed"=w387, "Right Drive Speed"=w390, "Lost Target Counter"=w397, "System State"=w394, "Spin Up Shooter Wheels"=TRUE) -> (w403:T5)
      }
      frame "Check for Stop" {
        # "As long as we have a distance calculation and\nits less than 20 feet we change states to stop"
        # "This checks the current robot position to determine if we need to stop driving towards target"
        n192 = Unbundle By Name(w412) -> ("Distance From Target"=w416:dbl, "System State"=w414:T1)
        n193 = Less?(x=w416, y=5.3) -> (x < y?=w417:bool)
        n194 = Not Equal To 0?(x=w416) -> (x != 0?=w418:bool)
        n195 = And(x=w418, y=w417) -> (x .and. y?=w406:bool)
        n196 = Select(t=AutomationDriveStates."Center Target", s=w406, f=w414) -> (s? t:f=w410:T1)
        n197 = Bundle By Name(cluster=w412, "System State"=w410) -> (w411:T5)
        n198 = Select(t="Center Target", s=w406, f="Drive Motors") -> (s? t:f=w407:string)
      }
      frame "Check for Restart" {
        # "Update Drive Time to maintain\ncurrent system state"
        # "Need to add code to determine when to restart searching algorithm"
        n199 = Unbundle By Name(w437) -> ("System State"=w436:T1)
        n200 = global read "Robot Global Data.vi" "Back Finger"() -> (w429:bool)
        n201 = global read "Robot Global Data.vi" "Front Finger"() -> (w430:bool)
        n202 = Select(t=WPI_SolenoidValue."Forward" ("Value"), s=w429, f=WPI_SolenoidValue."Reverse" ("Value")) -> (s? t:f=w419:T3)
        n203 = Select(t=WPI_SolenoidValue."Forward" ("Value"), s=w430, f=WPI_SolenoidValue."Reverse" ("Value")) -> (s? t:f=w420:T3)
        n204 = call <vilib>:"WPI_SolenoidRefNum Registry Get.vi"("refnum name"="shooterSolenoidForward") -> ("error out"=w421:errorcluster, "SolenoidDevRef"=w422:T30)  [unwired: 9 in]
        n205 = call <vilib>:"WPI_SolenoidRefNum Registry Get.vi"("refnum name"="shooterSolenoidBackward") -> ("error out"=w424:errorcluster, "SolenoidDevRef"=w425:T30)  [unwired: 9 in]
        n206 = call-poly <vilib>:"WPI_SolenoidSet.vi"("error in (no error)"=w421, "Value"=w420, "SolenoidDevRef"=w422) -> ()  [unwired: 7 in, 2 out]
        n207 = call-poly <vilib>:"WPI_SolenoidSet.vi"("error in (no error)"=w424, "Value"=w419, "SolenoidDevRef"=w425) -> ()  [unwired: 7 in, 2 out]
        n208 = Tick Count (ms)() -> (millisecond timer value=w434:u32)
        n209 = Bundle By Name(cluster=w437, "System State"=w436, "Last Drive Time"=w434, "In Position?"=FALSE) -> (w438:T5)
      }
      frame "Drive Motors" {
        w477 = 0.0 ("t")
        # "#When we decide on shooter \nmode put in the logic for changing\n the mode of the shooter"
        # "Store Last Drive Time to Track when Tele\nis disabled"
        # "Sends the Speed Targets to the Drive Motors"
        n210 = Unbundle By Name(w484) -> ("System State"=w482:T1, "Right Drive Speed"=w480:dbl, "Left Drive Speed"=w479:dbl, "Desired Arm State"=w476:T2, "Shoot"=w475:bool, "Spin Up Shooter Wheels"=w474:bool)
        n211 = call <vilib>:"WPI_MotorControlRefNum Registry Get.vi"("refnum name"="arm") -> ("MotorControlDevRef"=w467:T6)  [unwired: 9 in, 1 out]
        n212 = global read "Robot Global Data.vi" "Arm base offset"() -> (w470:dbl)
        n213 = call <vilib>:"WPI_CANTalonSRX_GetStatus.vi"("CAN Talon SRX Ref"=w467) -> ("Talon SRX Status"=w465:T28, "CAN Talon SRX Ref"=w464:T6)  [unwired: 8 in, 1 out]
        n214 = Unbundle By Name(w465) -> ("Pulse Width Position"=w462:i32)
        n215 = global read "Robot Global Data.vi" "Arm Power Vbus"() -> (w461:bool)
        n216 = Multiply(x=4095, y=3) -> (x*y=w471:i32)
        n217 = global read "Robot Global Data.vi" "Desired Arm Position"() -> (w460:dbl)
        n218 = Subtract(x=w471, y=w470) -> (x-y=w469:dbl)
        n219 = global read "Robot Global Data.vi" "Back Finger"() -> (w453:bool)
        n220 = global read "Robot Global Data.vi" "Front Finger"() -> (w454:bool)
        n221 = Equal?(x=AutomationDriveStates."Stop Drives", y=w482) -> (x = y?=w478:bool)
        n222 = global write "Robot Global Data.vi" "Desired Arm State From Auton"(w476) -> ()
        n223 = global write "Robot Global Data.vi" "Shoot From Auton"(w475) -> ()
        n224 = global write "Robot Global Data.vi" "Spin Up Wheels From Auton"(w474) -> ()
        n225 = Add(x=w462, y=w469) -> (x+y=w468:dbl)
        n226 = case shown="False" w461 {
          tunnel: [w491 w495] -> w463
          tunnel: w468 -> [_ w494]
          tunnel: w460 -> [w491 w492]
          frame True {
          }
          frame False {
            n227 = call-poly <vilib>:"PID.vi"("PID gains"=T4 {"proportional gain (Kc)"=0.0005, "integral time (Ti, min)"=0.0, "derivative time (Td, min)"=0.0}, "process variable"=w494, "setpoint"=w492) -> ("output"=w498:dbl)  [unwired: 7 in, 1 out]
            n228 = In Range and Coerce(upper limit=1.0, x=w498, lower limit=-1.0) -> (coerced(x)=w495:dbl)  [unwired: 1 out]
          }
        }
        n229 = Select(t=w477, s=w478, f=w480) -> (s? t:f=w442:dbl)
        n230 = Select(t=w477, s=w478, f=w479) -> (s? t:f=w441:dbl)
        n231 = Select(t=WPI_SolenoidValue."Forward" ("Value"), s=w453, f=WPI_SolenoidValue."Reverse" ("Value")) -> (s? t:f=w443:T3)
        n232 = Select(t=WPI_SolenoidValue."Forward" ("Value"), s=w454, f=WPI_SolenoidValue."Reverse" ("Value")) -> (s? t:f=w444:T3)
        n233 = Multiply(x=w441, y=1.0) -> (x*y=w440:dbl)
        n234 = call <vilib>:"WPI_MotorControlRefNum Registry Get.vi"("refnum name"="leftDrive") -> ("MotorControlDevRef"=w490:T6)  [unwired: 9 in, 1 out]
        n235 = call <vilib>:"WPI_MotorControlSetOutput.vi"("Output"=w440, "MotorControlDevRef"=w490) -> ()  [unwired: 7 in, 3 out]
        n236 = call <vilib>:"WPI_MotorControlSetOutput.vi"("Output"=w463, "MotorControlDevRef"=w464) -> ()  [unwired: 7 in, 3 out]
        n237 = call <vilib>:"WPI_SolenoidRefNum Registry Get.vi"("refnum name"="shooterSolenoidForward") -> ("error out"=w445:errorcluster, "SolenoidDevRef"=w446:T30)  [unwired: 9 in]
        n238 = call <vilib>:"WPI_SolenoidRefNum Registry Get.vi"("refnum name"="shooterSolenoidBackward") -> ("error out"=w448:errorcluster, "SolenoidDevRef"=w449:T30)  [unwired: 9 in]
        n239 = call-poly <vilib>:"WPI_SolenoidSet.vi"("error in (no error)"=w445, "Value"=w444, "SolenoidDevRef"=w446) -> ()  [unwired: 7 in, 2 out]
        n240 = call-poly <vilib>:"WPI_SolenoidSet.vi"("error in (no error)"=w448, "Value"=w443, "SolenoidDevRef"=w449) -> ()  [unwired: 7 in, 2 out]
        n241 = Tick Count (ms)() -> (millisecond timer value=w485:u32)
        n242 = call <vilib>:"WPI_MotorControlRefNum Registry Get.vi"("refnum name"="rightDrive") -> ("MotorControlDevRef"=w488:T6)  [unwired: 9 in, 1 out]
        n243 = global read "Robot Global Data.vi" "Shooter Speed"() -> (w457:dbl)
        n244 = call <vilib>:"WPI_MotorControlRefNum Registry Get.vi"("refnum name"="shooterWheel") -> ("MotorControlDevRef"=w458:T6)  [unwired: 9 in, 1 out]
        n245 = Bundle By Name(cluster=w484, "Last Drive Time"=w485) -> (w483:T5)
        n246 = call <vilib>:"WPI_MotorControlSetOutput.vi"("Output"=w442, "MotorControlDevRef"=w488) -> ()  [unwired: 7 in, 3 out]
        n247 = call <vilib>:"WPI_MotorControlSetOutput.vi"("Output"=w457, "MotorControlDevRef"=w458) -> ()  [unwired: 7 in, 3 out]
      }
      frame "Exit" {
      }
    }
  }
